vi "Climber_Hardware_Globals.vi"() -> ()   [LabVIEW 2020]
panel:
  in  "Outer_Arm_Limit_Switch":string="Outer_Arm_Limit_Switch"
  in  "Outer_Arm_Pivot_Brake_Pneumatic":string="Outer_Arm_Pivot_Brake_Pneumatic"
  in  "Elevator_Brake_Pneumatic":string="Elevator_Brake_Pneumatic"
  in  "Outer_Arm_Elevator_Right":string="Outer_Arm_Elevator_Right"
  in  "Outer_Arm_Elevator_Left":string="Outer_Arm_Elevator_Left"
  in  "Outer_Arm_Pivot":string="Outer_Arm_Pivot"
  in  "Inner_Arm_Pivot":string="Inner_Arm_Pivot"
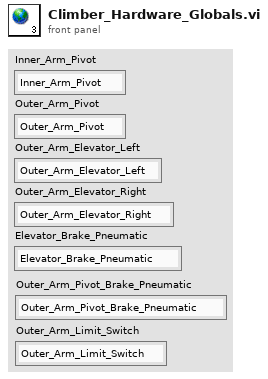
[diagram p1: front panel]
diagram:
